vi "Simulated Analog Data In.vi"(4 "error in (no error)":errorcluster, 7 "Plugin Name":T1) -> (0 "error out":errorcluster, 3 "Simulated Data":dbl)   [LabVIEW 2015, in "Startup Processes.lvlib"]
uses:
  Startup Processes.lvlib
  _typedefs/Subpanel Names.ctl
  <vilib>/ptbypt/NI_PtbyPt.lvlib
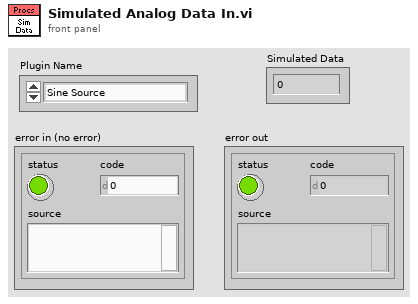
[diagram p1: front panel]
types:
  T1 = typedef "Startup Processes.lvlib/Subpanel Names.ctl" = enum16{"Sine Source", "Ramp Source", "Hen House TC", "Dog House TC", "Out House TC"}
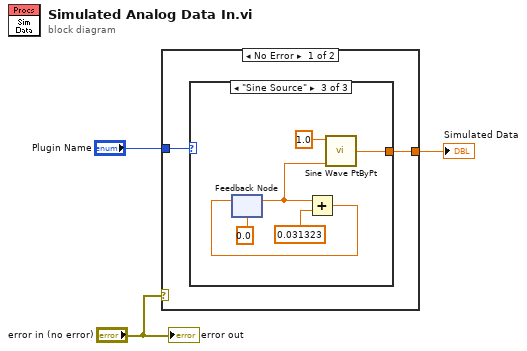
[diagram p0: block diagram]
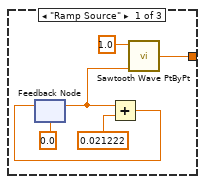
[diagram p2: hidden frame]
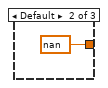
[diagram p3: hidden frame]
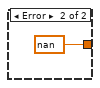
[diagram p4: hidden frame]
diagram:
  n1 = case shown="No Error" "error in (no error)" {
    tunnel: [w5 nan ("sawtooth wave")] -> w3
    tunnel: "Plugin Name" -> [w4 _]
    frame No Error {
      n2 = case shown="\"Sine Source\"" w4 {
        tunnel: [w11 nan ("sine wave") w13] -> w5
        frame "Ramp Source" {
          n3 = feedback #1(0.0) -> (w6:dbl)
          n4 = Add(x=w6, y=0.021222 ("amplitude")) -> (x+y=w7:dbl)
          n5 = feedback-in #1(w7) -> ()
          n6 = call <vilib>:"Sawtooth Wave PtByPt.vi"("time"=w6, "amplitude"=1.0) -> ("sawtooth wave"=w11:dbl)  [unwired: 2 in]
        }
        frame Default {
        }
        frame "Sine Source" {
          n7 = feedback #2(0.0) -> (w14:dbl)
          n8 = Add(x=w14, y=0.031323 ("amplitude")) -> (x+y=w16:dbl)
          n9 = feedback-in #2(w16) -> ()
          n10 = call <vilib>:"Sine Wave PtByPt.vi"("time"=w14, "amplitude"=1.0) -> ("sine wave"=w13:dbl)  [unwired: 2 in]
        }
      }
    }
    frame Error {
    }
  }
  "Simulated Data" <- w3
  "error out" <- "error in (no error)"
